vi "Init with Value.vi"(8 "error in":errorcluster, 10 "Value":variant, 11 "Cell in":refnum<class "Cell.lvclass">) -> (0 "error out":errorcluster, 3 "Cell out":refnum<class "Cell.lvclass">)   [LabVIEW 2024, in "SourceGrid.lvlib" / "Cell.lvclass"]
uses:
  Cell.lvclass
  Cell.lvclass/Cell.ctl
  D:/git/Sourcegrid-LabVIEW/dll/SourceGrid.dll
  dll/SourceGrid.dll
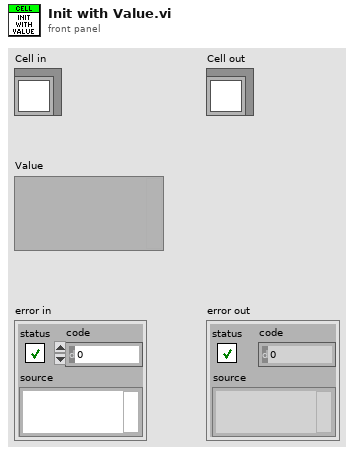
[diagram p1: front panel]
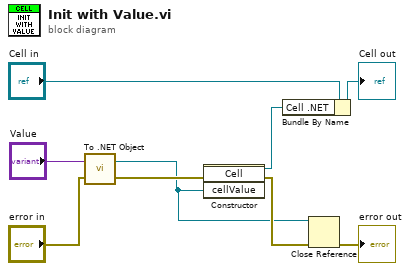
[diagram p0: block diagram]
diagram:
  n1 = call <vilib>:"To .NET Object.vi"("error in (no error)"="error in", "anything"="Value") -> ("error out"=w6:errorcluster, ".NET object"=w2:refnum<k24>)
  n2 = constructor class="Cell"(error in=w6, "cellValue"=w2) -> (reference out=w1:refnum<k24>, error out=w5:errorcluster)  [unwired: 2 in, 2 out]
  n3 = Bundle By Name(cluster="Cell in", "Cell .NET"=w1) -> (→"Cell out":refnum<class "Cell.lvclass">)
  n4 = Close Reference(reference=w2, error in (no error)=w5) -> (error out=→"error out":errorcluster)
